vi "Modbus_Init.vi"(8 "error in (no error)":errorcluster, 10 "Modbus RTU":T1={"unit ID"=1, "serial type"=enum."RTU", "baud rate"=9600, "parity (even)"=2, "flow control (none)"=0, "VISA resource name"=""} {"flow control (none)" items=["None", "XON/XOFF", "RTS/CTS", "XON/XOFF & RTS/CTS", "DTR/DSR", "XON/XOFF & DTR/DSR"]; "parity (even)" items=["None", "Odd", "Even", "Mark", "Space"]}, 11 "object in":refnum<class "Modbus.lvclass">) -> (0 "error out":errorcluster, 3 "object out":refnum<class "Modbus.lvclass">)   [LabVIEW 2023, in "HardwareAbstractionLayer_LVOOP.lvlib" / "Modbus.lvclass"]
uses:
  Modbus.lvclass
  <vilib>/NI/Modbus Library/API/Modbus API.lvclass/Modbus API.ctl
  <vilib>/NI/Modbus Library/Transmission Data Unit/Transmission Data Unit.lvclass/Transmission Data Unit.ctl
  Modbus.lvclass/Modbus.ctl
  <vilib>/NI/Modbus Library/API/Read Transmission Data Unit.vi
  <vilib>/NI/Modbus Library/API/Write Transmission Data Unit.vi
  <vilib>/NI/Modbus Library/Transmission Data Unit/Write read operation timeout.vi
  <vilib>/NI/Modbus Library/Transmission Data Unit/Write write operation timeout.vi
  <vilib>/NI/Modbus Library/API/Master/Modbus Master.lvclass
  <vilib>/NI/Modbus Library/API/Wrapper/Create Serial Master.vi
  <vilib>/NI/Modbus Library/API/Wrapper/API Main.lvlib
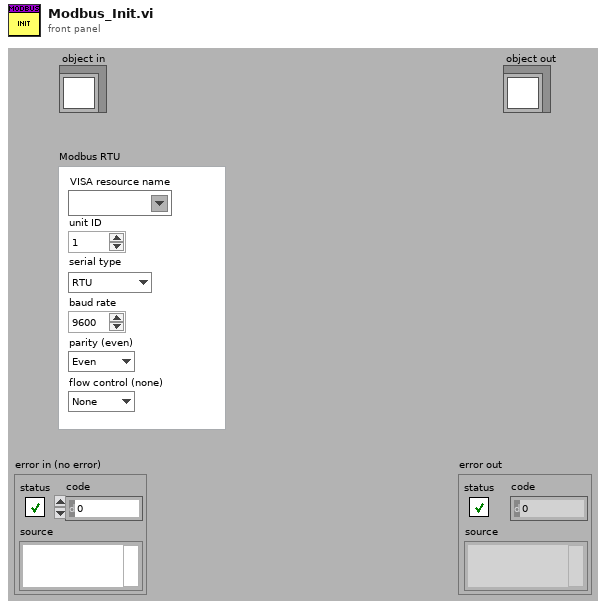
[diagram p1: front panel]
types:
  T1 = cluster{"unit ID":u8, "serial type":enum16{"RTU", "ASCII"}, "baud rate":u32, "parity (even)":u16, "flow control (none)":u16, "VISA resource name":refnum<visa-resource-name>}
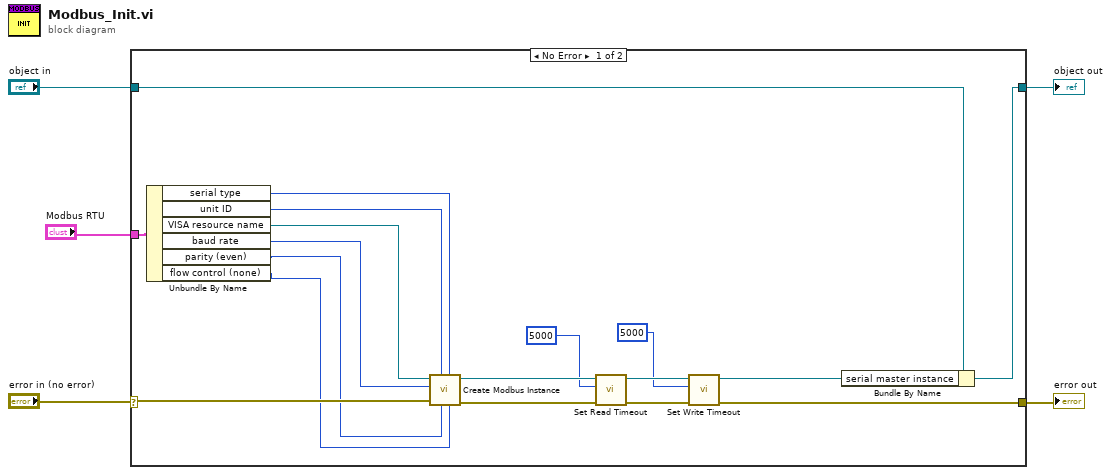
[diagram p0: block diagram]
diagram:
  n1 = case shown="No Error" "error in (no error)" {
    selector: "error in (no error)" -> [w21 w24]
    tunnel: "object in" -> [w22 w25]
    tunnel: [w23 w25] -> w4
    tunnel: [w10 w24] -> w2
    tunnel: "Modbus RTU" -> [w20 _]
    frame No Error {
      n2 = Unbundle By Name(w20) -> ("serial type"=w18:enum16{"RTU", "ASCII"}, "unit ID"=w17:u8, "VISA resource name"=w19:refnum<visa-resource-name>, "baud rate"=w16:u32, "parity (even)"=w15:u16, "flow control (none)"=w14:u16)
      n3 = call-poly <vilib>:"Create Modbus Instance.vi"("flow control (none)"=w14, "serial type"=w18, "parity (even)"=w15, "unit ID"=w17, "error in"=w21, "baud rate"=w16, "VISA resource name"=w19) -> ("error out"=w9:errorcluster, "serial master instance"=w13:refnum<class "Modbus Master.lvclass">)  [unwired: 3 in]
      n4 = call <vilib>:"Set Read Timeout.vi"("error in"=w9, "read operation timeout"=5000, "Modbus master in"=w13) -> ("error out"=w8:errorcluster, "Modbus master out"=w12:refnum<class "Modbus Master.lvclass">)  [unwired: 7 in]
      n5 = call <vilib>:"Set Write Timeout.vi"("error in"=w8, "write operation timeout"=5000, "Modbus master in"=w12) -> ("error out"=w10:errorcluster, "Modbus master out"=w11:refnum<class "Modbus Master.lvclass">)  [unwired: 7 in]
      n6 = Bundle By Name(cluster=w22, "serial master instance"=w11) -> (w23:refnum<class "Modbus.lvclass">)
    }
    frame Error {
    }
  }
  "object out" <- w4
  "error out" <- w2
